vi "Day 13-Combined x & y folds.vi"() -> ()   [LabVIEW 2021]
uses:
  <vilib>/Utility/file.llb/Read Delimited Spreadsheet (string).vi
  <vilib>/regexp/Match Regular Expression.xnode
panel:
  out "Array":bool[][](array[boolean])
  out "sum":i16
  out "subarray":string[](array[string])
  in  "Input File":enum32{"example input", "input"}(radio)
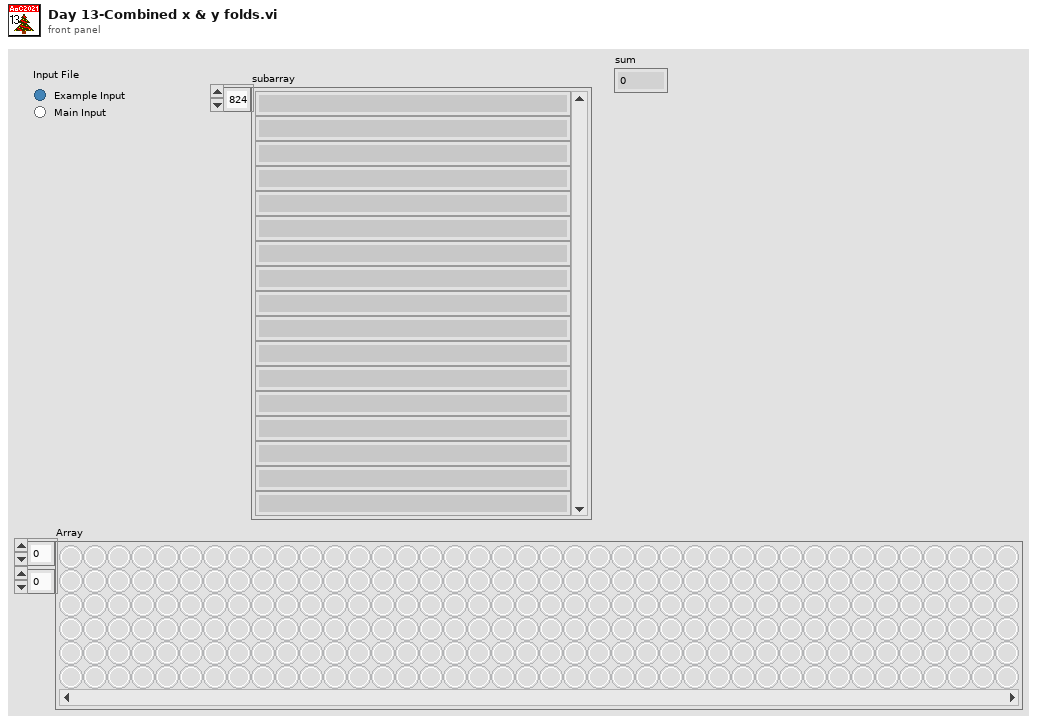
[diagram p1: front panel]
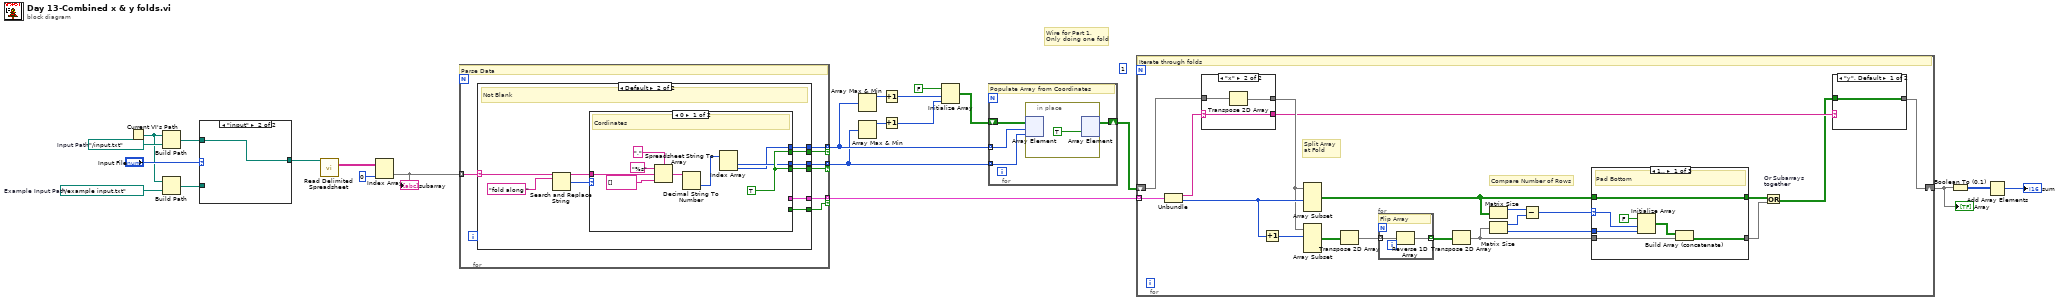
[diagram p0: block diagram]
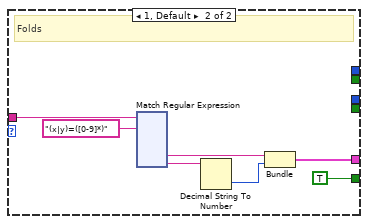
[diagram p3: hidden frame]
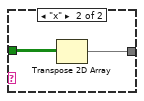
[diagram p5: hidden frame]
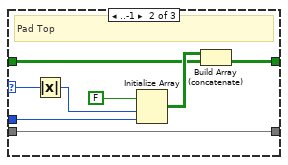
[diagram p7: hidden frame]
diagram:
  (unwired) 1
  w22 = path "../example input.txt"  # Example Input Path
  w23 = path "../input.txt"  # Input Path
  # "Wire for Part 1,\nOnly doing one fold"
  n1 = Current VI's Path() -> (path=w17:path)
  n2 = Build Path(base path=w17, name or relative path=w23) -> (appended path=w20:path)
  n3 = Build Path(base path=w17, name or relative path=w22) -> (appended path=w19:path)
  n4 = case shown="\"input\"" "Input File" {
    tunnel: w20 -> [_ w25]
    tunnel: w19 -> [w24 _]
    tunnel: [w24 w25] -> w18
    frame "example input" {
    }
    frame "input" {
    }
  }
  n5 = call-poly <vilib>:"Read Delimited Spreadsheet.vi"("file path (dialog if empty)"=w18) -> ("all rows"=w16:string[][])  [unwired: 9 in, 5 out]
  n6 = Index Array(array=w16, index (col)=0 ("disabled index (col)")) -> (element=w14:string[])  [unwired: 1 in]
  "subarray" <- w14
  n7 = for {
    tunnel: w14 -> [w32] mode=indexing
    tunnel: [w31] -> w13 mode=indexing if=w30
    tunnel: [w29] -> w5 mode=indexing if=w28
    tunnel: [w27] -> w12 mode=indexing if=w26
    # "Parse Data"
    n8 = case shown="Default" w32 {
      selector: w32 -> [_ w42]
      tunnel: [_ w38] -> w31
      tunnel: [_ w37] -> w30
      tunnel: [_ w36] -> w29
      tunnel: [_ w35] -> w28
      tunnel: [_ w34] -> w27
      tunnel: [_ w33] -> w26
      frame "" {
        # "Blank row"
      }
      frame Default {
        # "Not Blank"
        n9 = Search and Replace String(input string=w42, search string="fold along ") -> (result string=w39:string, number of replacements=w40:i32)  [unwired: 6 in, 2 out]
        n10 = case shown="0" w40 {
          tunnel: w39 -> [w51 w58]
          tunnel: [w43 _] -> w38
          tunnel: [w45 _] -> w37
          tunnel: [_ w53] -> w36
          tunnel: [_ TRUE] -> w35
          tunnel: [w44 _] -> w34
          tunnel: [w45 _] -> w33
          frame 0 {
            w45 = TRUE
            # "Cordinates"
            n11 = Spreadsheet String To Array(delimiter (Tab)=",", format string="%s", spreadsheet string=w51, array type (2D Dbl)=string[] []) -> (array=w47:string[])
            n12 = Decimal String To Number(string=w47) -> (number=w46:i32[])  [unwired: 2 in, 1 out]
            n13 = Index Array(array=w46) -> (element #1=w44:i32, element #2=w43:i32)  [unwired: 2 in]
          }
          frame 1, Default {
            # "Folds"
            n14 = xnode "Match Regular Expression"("input string"=w58, "regular expression"="(x|y)=([0-9]*)") -> ("submatch 1"=w55:string, "submatch 2"=w56:string)  [unwired: 4 in, 5 out]
            n15 = Decimal String To Number(string=w56) -> (number=w54:i32)  [unwired: 2 in, 1 out]
            n16 = Bundle("submatch 1"=w55, w54) -> (w53:cluster{"submatch 1":string, i32})  [unwired: 1 in]
          }
        }
      }
    }
  }
  n17 = Array Max & Min(array=w13) -> (max value=w11:i32)  [unwired: 3 out]
  n18 = Array Max & Min(array=w12) -> (max value=w8:i32)  [unwired: 3 out]
  n19 = Increment(x=w11) -> (x+1=w9:i32)
  n20 = Increment(x=w8) -> (x+1=w7:i32)
  n21 = Initialize Array(FALSE, w9, w7) -> (w6:bool[][])
  n22 = for {
    tunnel: w13 -> [w181] mode=indexing
    tunnel: w12 -> [w180] mode=indexing
    shift-right: [w179] -> w4
    shift-left: w6 -> [w182]
    # "Populate Array from Coordinates"
    n23 = in-place {
      n24 = in-place-array #1(w182, w181, w180) -> ()  [unwired: 1 out]
      n25 = in-place-array #1(TRUE) -> (w179:bool[][])  [unwired: 2 out]
    }
  }
  n26 = for {
    tunnel: w5 -> [w203] mode=indexing
    shift-right: [w184] -> w3
    shift-left: w4 -> [w189]
    # "Compare Number of Rows"
    # "Split Array at Fold"
    # "Iterate through folds"
    n27 = Unbundle(w203) -> ("submatch 1"=w187:string, w202:i32)
    n28 = case shown="\"x\"" w187 {
      selector: w187 -> [w207 w209]
      tunnel: w189 -> [w208 w211]
      tunnel: [w208 w210] -> w188
      tunnel: [w207 w209] -> w186
      frame "y", Default {
      }
      frame "x" {
        n29 = Transpose 2D Array(2D array=w211) -> (transposed array=w210:bool[][])
      }
    }
    n30 = Increment(x=w202) -> (x+1=w200:i32)
    n31 = Array Subset(array=w188, length (row)=w202) -> (w193:bool[][])  [unwired: 3 in]
    n32 = Array Subset(array=w188, index (row)=w200) -> (w201:bool[][])  [unwired: 3 in]
    n33 = Transpose 2D Array(2D array=w201) -> (transposed array=w199:bool[][])
    n34 = for {
      tunnel: w199 -> [w230] mode=indexing
      tunnel: [w229] -> w198 mode=indexing
      # "Flip Array"
      n35 = Reverse 1D Array(array=w230) -> (reversed array=w229:bool[])
    }
    n36 = Transpose 2D Array(2D array=w198) -> (transposed array=w191:bool[][])
    n37 = Matrix Size(0:w193) -> (1:w197:i32)  [unwired: 1 out]
    n38 = Matrix Size(0:w191) -> (1:w196:i32, 2:w190:i32)
    n39 = Subtract(x=w197, y=w196) -> (x-y=w195:i32)
    n40 = case shown="1.." w195 {
      selector: w195 -> [w217 w225 _]
      tunnel: [w212 w222 w228] -> w194
      tunnel: w193 -> [w212 w221 w228]
      tunnel: [w213 w220 w227] -> w192
      tunnel: w191 -> [w214 w220 w227]
      tunnel: w190 -> [w216 w224 _]
      frame 1.. {
        # "Pad Bottom"
        n41 = Initialize Array(FALSE, w217, w216) -> (w215:bool[][])
        n42 = Build Array (concatenate)(w215, w214) -> (w213:bool[][])
      }
      frame ..-1 {
        # "Pad Top"
        n43 = Absolute Value(x=w225) -> (abs(x)=w219:i32)
        n44 = Initialize Array(FALSE, w219, w224) -> (w223:bool[][])
        n45 = Build Array (concatenate)(w223, w221) -> (w222:bool[][])
      }
      frame 0 {
        # "Same Size"
      }
    }
    n46 = Or "Or Subarrays\ntogether"(x=w194, y=w192) -> (x .or. y?=w185:bool[][])
    n47 = case shown="\"y\", Default" w186 {
      tunnel: w185 -> [w204 w206]
      tunnel: [w204 w205] -> w184
      frame "y", Default {
      }
      frame "x" {
        n48 = Transpose 2D Array(2D array=w206) -> (transposed array=w205:bool[][])
      }
    }
  }
  "Array" <- w3
  n49 = Boolean To (0,1)(Boolean=w3) -> (0, 1=w2:i16[][])
  n50 = Add Array Elements(numeric array=w2) -> (sum=→"sum":i16)
